vi "Emballage_BDD check code lu.vi"(2 "error in":errorcluster caption="entrée d'erreur", 3 "n° lot à scanner":string="0808", 4 "chaîne lue par le lecteur IN":string="112105740008090004", 5 "tab pcs déjà emballées (histo+actu)":string[](array[string])=["112105740008090009", "112105740008090004", "112105740008090006", "112105740008090007", "112105740008090007R1"], 6 "Quantité du lot de livraison":i32, 16 "n° commande EC":string="R03838/08-01.01.01") -> (9 "error out":errorcluster caption="sortie d'erreur", 13 "offset sur code bar début index":i16=-1, 14 "largeur index":i16=-1, 15 "Date production de la piéce":string, 17 "chaîne lue par le lecteur OUT":string="112105740008090004R1", 18 "Arrêter la série (T)":bool, 19 "Paramètres OK(=> T)":bool)   [LabVIEW 2020]
uses:
  Modules/FS/60_FS_Controles/60_FS_SetGet.ctl
  VG_VerifTests_ModeRetour.vi
  Instance           3 31Saved   Emballage check code lu .vi
panel:
  out "Glissière 2":u8(slide)=100 caption="Identification terminé." scale=0.0..100.0
  out "RETOUR CLIENT":string="1"
  out "tab pcs emballées historique":string[][](array[string])=[["112105740008090004", "01.01.2001 01:01:00", "55", "01234/08-01.01.01", "1", "0"], ["112105740008090006", "01.01.2001 01:01:00", "55", "56789/08-01.01.01", "3", "0"], ["112105740008090007", "01.01.2001 01:01:00", "55", "56789/08-01.01.01", "4", "0"], ["112105740008090007", "01.01.2001 01:01:00", "55", "00123/08-01.01.01", "2", "1"]]
  # "dans historique :\ncolonne 0 = numéro de pièce\ncolonne 1 = date\ncolonne 2 = visa emball\ncolonne 3 = No commande\ncolonne 4 = carton\ncolonne 5 = qtté cmdée ou RC"
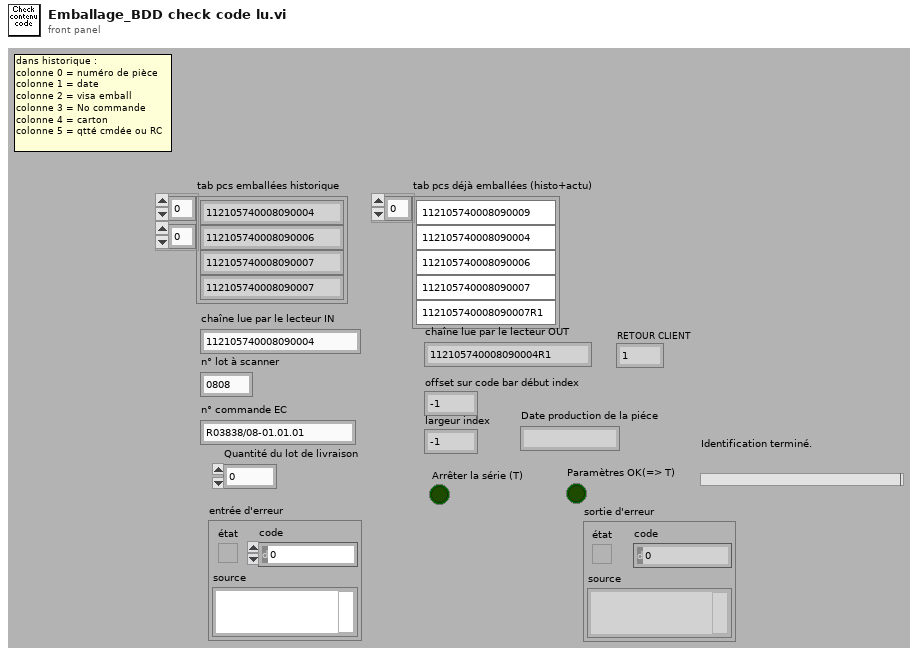
[diagram p1: front panel]
types:
  T1 = typedef "60_FS_SetGet.ctl" = enum16{"set", "get"}
  T2 = typedef "Emballage_BDD_param_Produit.ctl" = cluster{"No_Valve_FAS":string, "suffixe":string, "designation":string, "indice_produit":string, "code_barre_fixe":string, "affiche_code_barre_client":string, "affiche_no_client":string, "Nb_vlve_par_carton":u16, "melange_des_lots_possible":string, "id_article":string, "Indice_Rev":string, "Famille":string, "date":string, "code_barre_fixe_Fin":string, "Longeur_No_Serie":string}
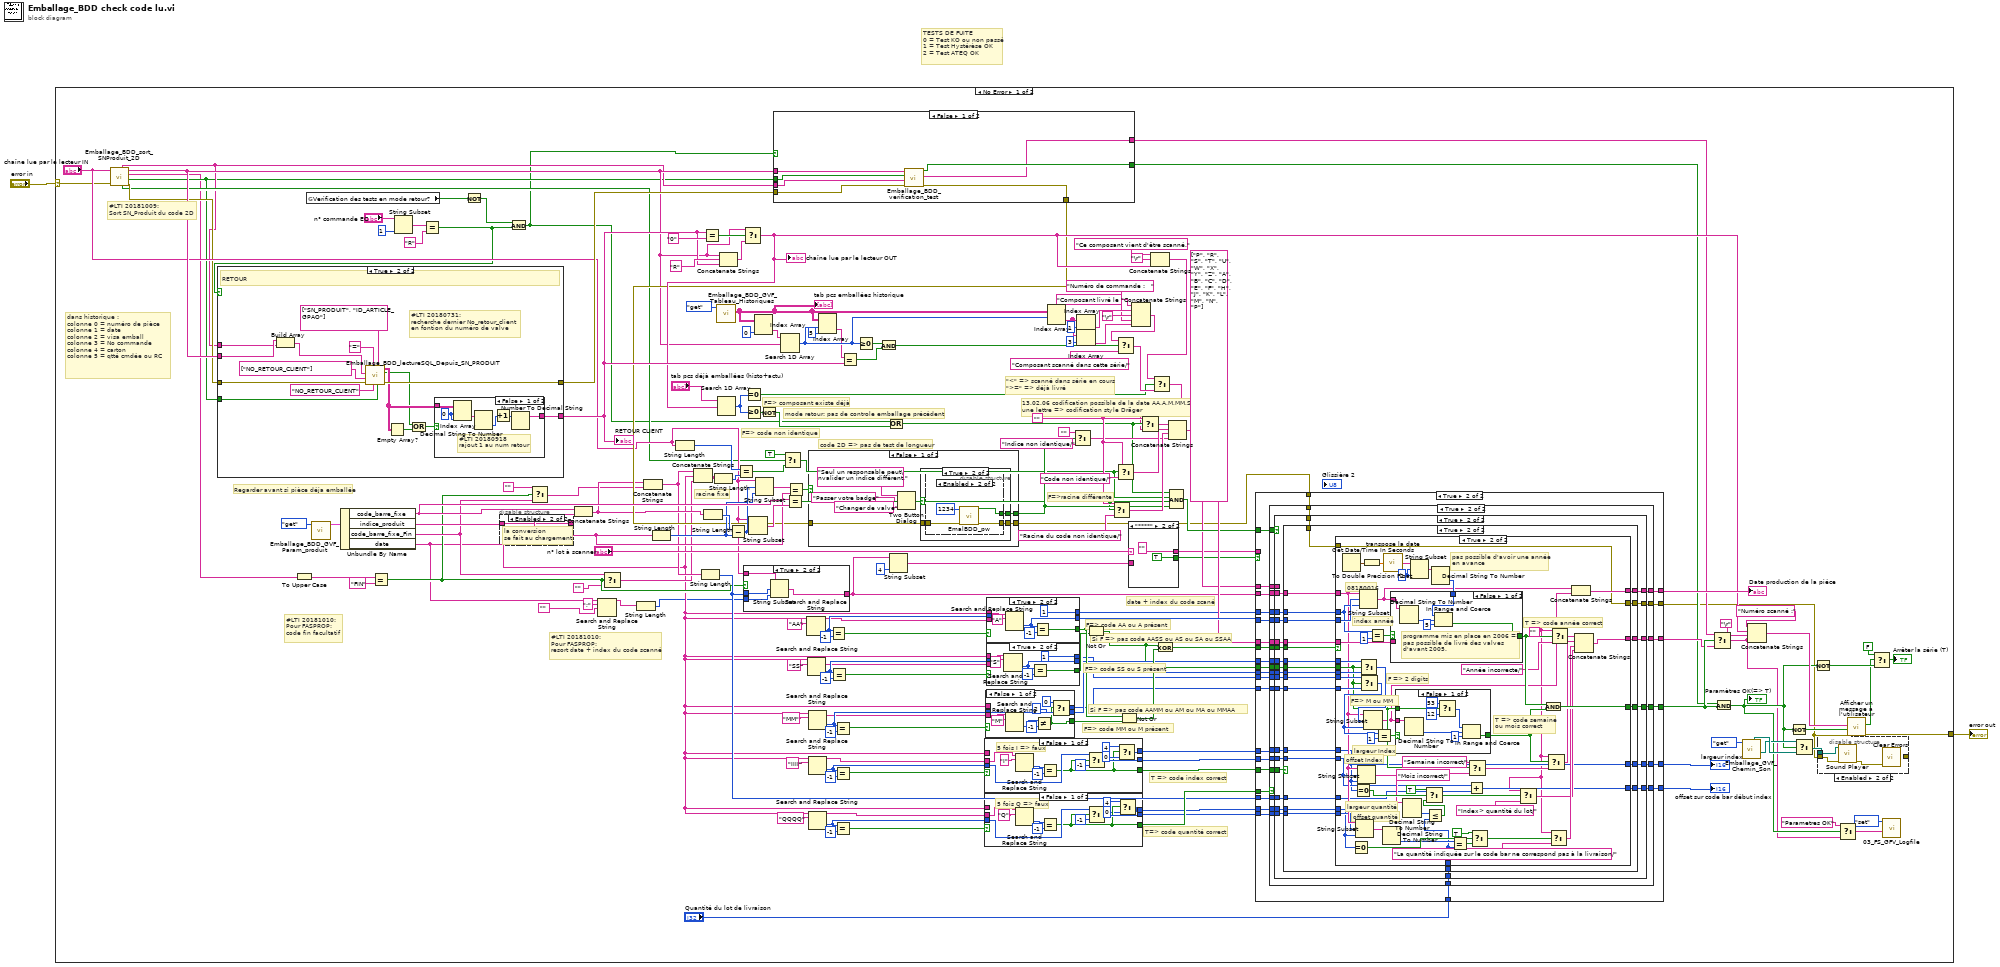
[diagram p0: block diagram]
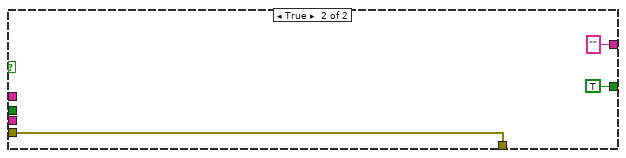
[diagram p2: hidden frame]
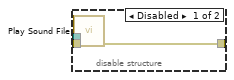
[diagram p3: hidden frame]
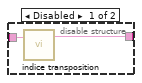
[diagram p4: hidden frame]
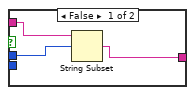
[diagram p5: hidden frame]
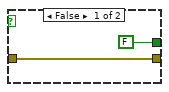
[diagram p6: hidden frame]
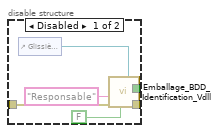
[diagram p7: hidden frame]
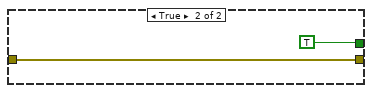
[diagram p8: hidden frame]
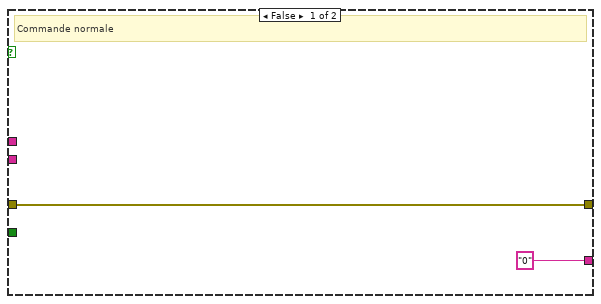
[diagram p9: hidden frame]
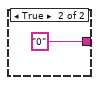
[diagram p10: hidden frame]
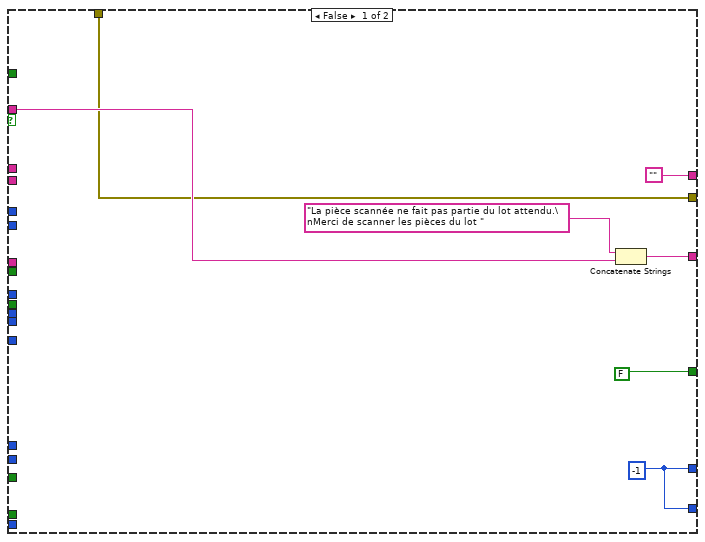
[diagram p11: hidden frame]
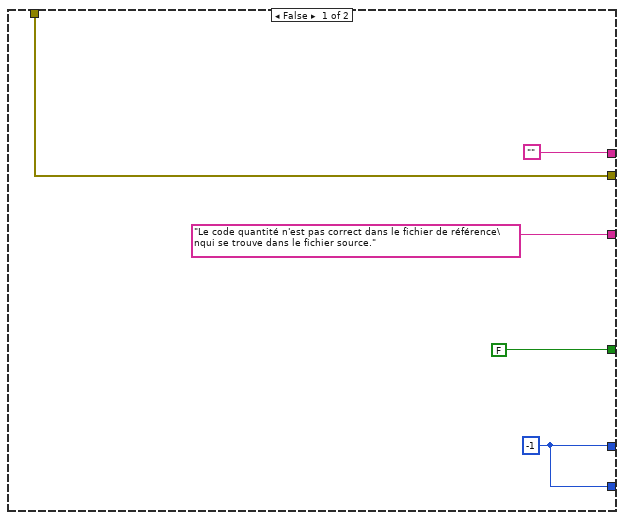
[diagram p12: hidden frame]
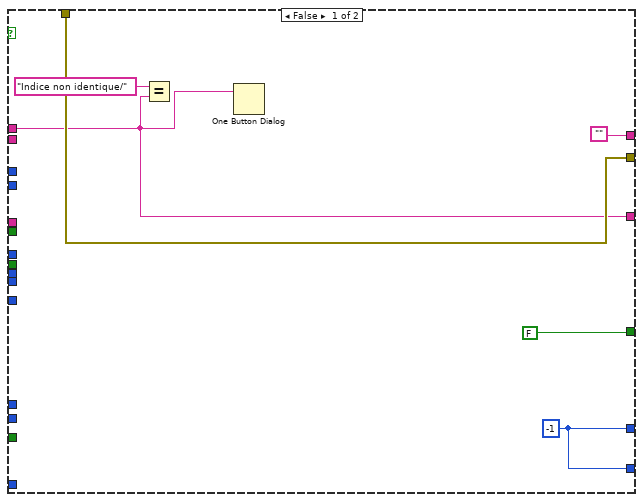
[diagram p13: hidden frame]
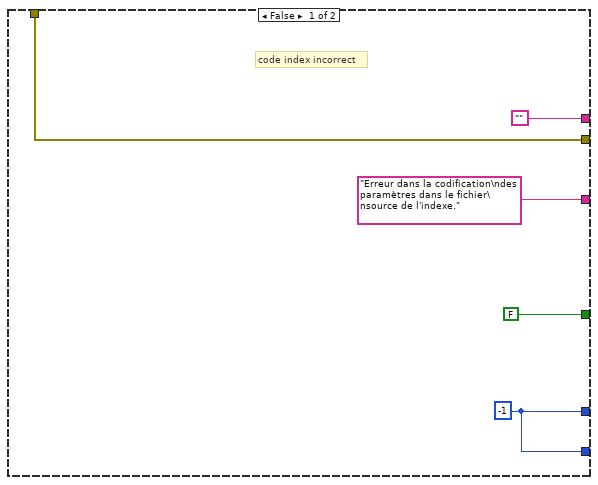
[diagram p14: hidden frame]
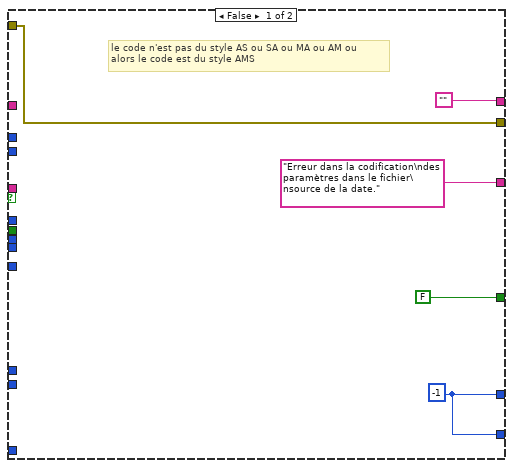
[diagram p15: hidden frame]
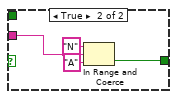
[diagram p16: hidden frame]
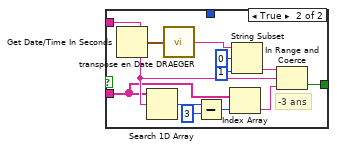
[diagram p17: hidden frame]
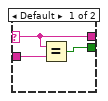
[diagram p18: hidden frame]
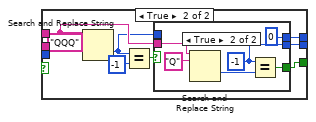
[diagram p19: hidden frame]
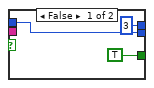
[diagram p20: hidden frame]
diagram:
  # "TESTS DE FUITE\n0 = Test KO ou non passé\n1 = Test Hystérèse OK\n2 = Test ATEQ OK"
  n1 = case shown="No Error" "error in" {
    selector: "error in" -> [w33 w580]
    tunnel: [w70 w580] -> w1
    frame No Error {
      w145 = ""
      # "code 2D => pas de test de longueur"
      # "#LTI 20181010:\nPour FASPROP:\nresort date + index du code scanné"
      # "#LTI 20181010:\nPour FASPROP:\ncode fin facultatif"
      # "#LTI 20181009:\nSort SN_Produit du code 2D"
      # "mode retour: pas de controle emballage précédent"
      # "Regarder avant si pièce déja emballée"
      # "dans historique :\ncolonne 0 = numéro de pièce\ncolonne 1 = date\ncolonne 2 = visa emball\ncolonne 3 = No commande\ncolonne 4 = carton\ncolonne 5 = qtté cmdée ou RC"
      # "\"<\" => scanné dans série en cours\n\">=\" => déjà livré"
      # "T=> code quantité correct"
      # "Si F => pas code AASS ou AS ou SA ou SSAA"
      # "Si F => pas code AAMM ou AM ou MA ou MMAA"
      # "F=> code MM ou M présent"
      # "F=> code SS ou S présent"
      # "F=> code AA ou A présent"
      # "T => code index correct"
      # "13.02.06 codification possible de la date AA,A,M,MM,S,SS\nune lettre => codification style Dräger"
      # "date + index du code scané"
      # "racine fixe"
      # "F=> composant existe déjà"
      # "F=> code non identique"
      # "F=>racine différente"
      n2 = call "Emballage_BDD_sort_SNProduit_2D.vi"("Error in"=w33, "Chaine_Lecteur"="chaîne lue par le lecteur IN") -> ("Error out"=w32:errorcluster, "ID_ARTICLE?"=w12:bool, "emplacement_CodeBarreFinFixe"=w11:string, "SN_PRODUIT"=w36:string, "Code 2D?"=w18:bool, "ID_ARTICLE"=w13:string)  [unwired: 4 in]
      n3 = To Upper Case(1:w11) -> (0:w30:string)
      n4 = global read "VG_VerifTests_ModeRetour.vi" "Verification des tests en mode retour?"() -> (w49:bool)
      n5 = call "Emballage_BDD_GVF_Param_produit.vi"("Énum"=enum16{"set", "get"}."get") -> ("CLS_param_produit"=w43:T2)  [unwired: 7 in, 3 out]
      n6 = Unbundle By Name(w43) -> ("code_barre_fixe"=w64:string, "indice_produit"=w63:string, "code_barre_fixe_Fin"=w26:string, "date"=w23:string)
      n7 = Equal?(x=w30, y="FIN") -> (x = y?=w25:bool)
      n8 = String Subset(string="n° commande EC", length (rest)=1 ("longueur (reste)")) -> (substring=w83:string)  [unwired: 1 in]
      n9 = Equal?(x=w83, y="R" ("expression régulière")) -> (x = y?=w4:bool)
      n10 = case shown="True" w4 {
        tunnel: w36 -> [_ w248]
        tunnel: ["0" ("expression régulière") w247] -> w73
        tunnel: w32 -> [w232 w246]
        tunnel: [w232 w245] -> w69
        tunnel: w13 -> [_ w244]
        tunnel: w12 -> [_ w243]
        frame False {
          # "Commande normale"
        }
        frame True {
          # "#LTI 20180731:\nrecherche dernier No_retour_client\nen fontion du numéro de valve"
          # "RETOUR"
          n11 = Build Array(w248, w244) -> (w235:string[])
          n12 = call "Emballage_BDD_lectureSQL_Depuis_SN_PRODUIT.vi"("ID_ARTICLE?"=w243, "Where (Champs:SN_PRODUIT)"=string[] ["SN_PRODUIT", "ID_ARTICLE_GPAO"], "order by ... DESC"="NO_RETOUR_CLIENT" ("order by"), "Where (Like/=)"="=", "Error in"=w246, "Colonnes"=string[] ["NO_RETOUR_CLIENT"], "Where (Valeur)"=w235) -> ("Error out"=w245:errorcluster, "Erreur de  comunication"=w234:bool, "Donnees"=w239:string[][])  [unwired: 2 in]
          n13 = Empty Array?(array=w239) -> (empty?=w237:bool)
          n14 = Or(x=w234, y=w237) -> (x .or. y?=w238:bool)
          n15 = case shown="False" w238 {
            tunnel: [w249 "0" ("String")] -> w247
            tunnel: w239 -> [w253 _]
            frame False {
              w254 = 0 ("indice (ligne)")
              # "#LTI 20180918\nrajout 1 au num retour"
              n16 = Index Array(array=w253, index (row)=w254, index (col)=w254) -> (element=w252:string)
              n17 = Decimal String To Number(string=w252) -> (number=w251:i32)  [unwired: 2 in, 1 out]
              n18 = Increment(x=w251) -> (x+1=w250:i32)
              n19 = Number To Decimal String(number=w250) -> (decimal integer string=w249:string)  [unwired: 1 in]
            }
            frame True {
            }
          }
        }
      }
      "RETOUR CLIENT" <- w73
      n20 = Not(x=w49) -> (.not. x?=w48:bool)
      n21 = disable-structure shown="Enabled" {
        disable-tunnel: w63 -> [w199 w200]
        disable-tunnel: [w198 w200] -> w59
        frame Disabled {
          n22 = call "indice transposition.vi"("indice entrée"=w199) -> ("indice corrigé"=w198:string)  [unwired: 1 in, 1 out]
        }
        frame Enabled {
          # "la conversion \nse fait au chargement"
        }
      }
      n23 = And(x=w48, y=w4) -> (x .and. y?=w3:bool)
      n24 = Select(t="", s=w25, f=w26) -> (s? t:f=w29:string)
      n25 = Concatenate Strings(w64, w59) -> (w39:string)
      n26 = Search and Replace String(input string=w23, search string=";" ("chaîne recherchée"), replace string="") -> (result string=w20:string)  [unwired: 5 in, 3 out]
      n27 = Select(t=w26, s=w25, f="") -> (s? t:f=w27:string)
      n28 = String Length(string=w20) -> (length=w19:i32)
      n29 = Concatenate Strings(w39, w29) -> (w38:string)
      n30 = String Length(string=w59) -> (length=w61:i32)
      n31 = String Length(string="chaîne lue par le lecteur IN") -> (length=w180:i32)
      n32 = Concatenate Strings(w38, w23, w27) -> (w181:string)
      n33 = String Length(string=w38) -> (length=w37:i32)
      n34 = Equal?(x=w73, y="0" ("chaîne")) -> (x = y?=w74:bool)
      n35 = String Length(string=w39) -> (length=w65:i32)
      n36 = String Length(string=w181) -> (length=w179:i32)
      n37 = call "Emballage_BDD_GVF_Tableau_Historiques.vi"("SetGet"=60_FS_SetGet."get") -> ("Tableau historique OUT"=w42:string[][])  [unwired: 9 in, 1 out]
      "tab pcs emballées historique" <- w42
      n38 = Concatenate Strings(w36, "R" ("chaîne"), w73) -> (w72:string)
      n39 = Subtract(x=w65, y=w61) -> (x-y=w62:i32)
      n40 = Equal?(x=w180, y=w179) -> (x = y?=w17:bool)
      n41 = Select(t=w36, s=w74, f=w72) -> (s? t:f=w71:string)
      "chaîne lue par le lecteur OUT" <- w71
      n42 = Search 1D Array(1D array="tab pcs déjà emballées (histo+actu)", element=w71) -> (index of element=w102:i32)  [unwired: 1 in]
      n43 = case shown="True" w25 {
        tunnel: [w203 w204] -> w95
        tunnel: w37 -> [w202 w206]
        tunnel: "chaîne lue par le lecteur IN" -> [w201 w207]
        tunnel: w19 -> [_ w205]
        frame False {
          n44 = String Subset(string=w201, offset (0)=w202) -> (substring=w203:string)  [unwired: 1 in]
        }
        frame True {
          n45 = String Subset(string=w207, offset (0)=w206, length (rest)=w205) -> (substring=w204:string)
        }
      }
      n46 = Equal To 0?(x=w102) -> (x = 0?=w100:bool)
      n47 = Greater Or Equal To 0?(x=w102) -> (x >= 0?=w149:bool)
      n48 = String Subset(string="chaîne lue par le lecteur IN", length (rest)=w62) -> (substring=w178:string)  [unwired: 1 in]
      n49 = Index Array(array=w42, index (col)=0) -> (element=w103:string[])  [unwired: 1 in]
      n50 = String Subset(string="chaîne lue par le lecteur IN", offset (0)=w62, length (rest)=w61) -> (substring=w60:string)
      n51 = Not(x=w149) -> (.not. x?=w148:bool)
      n52 = case shown="False" w3 {
        tunnel: w36 -> [w188 _]
        tunnel: w69 -> [w187 w189]
        tunnel: [w186 w189] -> w54
        tunnel: [w185 TRUE ("résultat_valve")] -> w50
        tunnel: [w184 "" ("Chaîne explique_probleme")] -> w66
        tunnel: w12 -> [w183 _]
        tunnel: w13 -> [w182 _]
        frame False {
          n53 = call "Emballage_BDD_verification_test.vi"("Error in"=w187, "ID_ARTICLE"=w182, "ID_ARTICLE?"=w183, "Piece_Scanne"=w188) -> ("Error out"=w186:errorcluster, "Chaîne explique_probleme"=w184:string, "résultat_valve"=w185:bool)  [unwired: 5 in]
        }
        frame True {
        }
      }
      n54 = Search 1D Array(1D array=w103, element=w36) -> (index of element=w82:i32)  [unwired: 1 in]
      n55 = Select(t=TRUE ("cas vrai"), s=w18, f=w17) -> (s? t:f=w16:bool)
      n56 = Equal?(x=w64, y=w178) -> (x = y?=w34:bool)
      n57 = Equal?(x=w60, y=w59) -> (x = y?=w55:bool)
      n58 = Search and Replace String(input string=w23, search string="AA") -> (result string=w139:string, offset past replacement=w165:i32)  [unwired: 6 in, 2 out]
      n59 = Search and Replace String(input string=w23, search string="SS") -> (result string=w125:string, offset past replacement=w164:i32)  [unwired: 6 in, 2 out]
      n60 = case shown="False" w55 {
        tunnel: w54 -> [w214 w231]
        tunnel: [w213 w231] -> w53
        tunnel: [w212 TRUE] -> w52
        frame False {
          n61 = Two Button Dialog(message="Seul un responsable peut\nvalider un indice différent.", 1:"Changer de valve" ("Nom du bouton F (\"Annuler\")"), 2:"Passer votre badge" ("Nom du bouton V (\"OK\")")) -> (T button?=w211:bool)
          n62 = case shown="True" w211 {
            tunnel: w214 -> [w216 w219]
            tunnel: [w216 w218] -> w213
            tunnel: [FALSE ("OK") w217] -> w212
            frame False {
            }
            frame True {
              n63 = disable-structure shown="Enabled" {
                disable-tunnel: w219 -> [w222 w228]
                disable-tunnel: [w221 w227] -> w218
                disable-tunnel: [w220 w226] -> w217
                frame Disabled {
                  n64 = control-ref of="Glissière 2"() -> (w225:refnum<vi>)
                  n65 = call "Emballage_BDD_Identification_Vdll.vi"("Glissière"=w225, "lecture seul possible ?"=FALSE, "error in"=w222, "Posage choisi"="Responsable" ("Posage choissi")) -> ("error Out"=w221:errorcluster, "OK"=w220:bool)  [unwired: 3 in, 3 out]
                }
                frame Enabled {
                  n66 = call "EmalBDD_pw.vi"("Error in"=w228, "PWattendu"=u32 1234) -> ("Error Out"=w227:errorcluster, "pwOK?"=w226:bool)  [unwired: 8 in]
                }
              }
            }
          }
        }
        frame True {
        }
      }
      n67 = Search and Replace String(input string=w23, search string="MM") -> (result string=w124:string, offset past replacement=w163:i32)  [unwired: 6 in, 2 out]
      n68 = Search and Replace String(input string=w23, search string="IIII") -> (result string=w140:string, offset past replacement=w134:i32)  [unwired: 6 in, 2 out]
      n69 = Search and Replace String(input string=w23, search string="QQQQ") -> (result string=w132:string, offset past replacement=w131:i32)  [unwired: 6 in, 2 out]
      n70 = Index Array(array=w42, index (row)=w82, index (col)=5) -> (element=w80:string)
      n71 = Equal?(x=w165, y=-1) -> (x = y?=w170:bool)
      n72 = Equal?(x=w164, y=-1) -> (x = y?=w171:bool)
      n73 = Equal?(x=w163, y=-1) -> (x = y?=w169:bool)
      n74 = Equal?(x=w134, y=-1) -> (x = y?=w166:bool)
      n75 = Equal?(x=w131, y=-1) -> (x = y?=w126:bool)
      n76 = Equal?(x=w80, y=w73) -> (x = y?=w79:bool)
      n77 = Greater Or Equal To 0?(x=w82) -> (x >= 0?=w78:bool)
      n78 = And(x=w78, y=w79) -> (x .and. y?=w77:bool)
      n79 = Or(x=w3, y=w148) -> (x .or. y?=w51:bool)
      n80 = String Subset(string=w95, length (rest)=4 ("longueur (reste)")) -> (substring=w90:string)  [unwired: 1 in]
      n81 = case shown="False" w166 {
        tunnel: w23 -> [_ w520]
        tunnel: [w506 w519] -> w135
        tunnel: w140 -> [w512 _]
        tunnel: w134 -> [w511 _]
        tunnel: [w509 w517] -> w133
        tunnel: [w505 w516] -> w128
        frame False {
          # "5 fois I => faux"
          n82 = Search and Replace String(input string=w512, search string="I") -> (offset past replacement=w513:i32)  [unwired: 6 in, 3 out]
          n83 = Equal?(x=w513, y=-1) -> (x = y?=w506:bool)
          n84 = Select(t=w511, s=w506, f=-1) -> (s? t:f=w509:i32)
          n85 = Select(t=4, s=w506, f=0) -> (s? t:f=w505:i32)
        }
        frame True {
          n86 = Search and Replace String(input string=w520, search string="III") -> (offset past replacement=w518:i32)  [unwired: 6 in, 3 out]
          n87 = Equal?(x=w518, y=-1) -> (x = y?=w521:bool)
          n88 = case shown="True" w521 {
            tunnel: w520 -> [_ w531]
            tunnel: [TRUE w529] -> w519
            tunnel: w518 -> [w525 _]
            tunnel: [w525 w528] -> w517
            tunnel: [3 0] -> w516
            frame False {
            }
            frame True {
              w528 = -1
              n89 = Search and Replace String(input string=w531, search string="I") -> (offset past replacement=w530:i32)  [unwired: 6 in, 3 out]
              n90 = Equal?(x=w528, y=w530) -> (x = y?=w529:bool)
            }
          }
        }
      }
      n91 = case shown="False" w126 {
        tunnel: w23 -> [_ w492]
        tunnel: [w480 w491] -> w130
        tunnel: w132 -> [w484 _]
        tunnel: w131 -> [w483 _]
        tunnel: [w481 w489] -> w129
        tunnel: [w477 w488] -> w127
        frame False {
          # "5 fois Q => faux"
          n92 = Search and Replace String(input string=w484, search string="Q") -> (offset past replacement=w485:i32)  [unwired: 6 in, 3 out]
          n93 = Equal?(x=w485, y=-1) -> (x = y?=w480:bool)
          n94 = Select(t=w483, s=w480, f=-1) -> (s? t:f=w481:i32)
          n95 = Select(t=4, s=w480, f=0) -> (s? t:f=w477:i32)
        }
        frame True {
          n96 = Search and Replace String(input string=w492, search string="QQQ") -> (offset past replacement=w490:i32)  [unwired: 6 in, 3 out]
          n97 = Equal?(x=w490, y=-1) -> (x = y?=w493:bool)
          n98 = case shown="True" w493 {
            tunnel: w492 -> [_ w503]
            tunnel: [TRUE w501] -> w491
            tunnel: w490 -> [w497 _]
            tunnel: [w497 w500] -> w489
            tunnel: [3 0] -> w488
            frame False {
            }
            frame True {
              w500 = -1
              n99 = Search and Replace String(input string=w503, search string="Q") -> (offset past replacement=w502:i32)  [unwired: 6 in, 3 out]
              n100 = Equal?(x=w500, y=w502) -> (x = y?=w501:bool)
            }
          }
        }
      }
      n101 = case shown="False" w169 {
        tunnel: w23 -> [_ w547]
        tunnel: [w534 w544] -> w162
        tunnel: [w541 w543] -> w155
        tunnel: w163 -> [w541 _]
        tunnel: [w536 1] -> w152
        tunnel: w124 -> [w537 _]
        frame False {
          n102 = Search and Replace String(input string=w537, search string="M") -> (offset past replacement=w540:i32)  [unwired: 6 in, 3 out]
          n103 = Not Equal?(x=w540, y=-1) -> (x != y?=w534:bool)
          n104 = Select(t=0, s=w534, f=2) -> (s? t:f=w536:i32)
        }
        frame True {
          n105 = Search and Replace String(input string=w547, search string="M") -> (offset past replacement=w543:i32)  [unwired: 6 in, 3 out]
          n106 = Equal?(x=w543, y=-1) -> (x = y?=w544:bool)
        }
      }
      n107 = case shown="True" w171 {
        tunnel: w23 -> [_ w562]
        tunnel: w164 -> [w556 _]
        tunnel: [w556 w559] -> w156
        tunnel: [w548 w558] -> w160
        tunnel: [w551 1] -> w153
        tunnel: w125 -> [w552 _]
        frame False {
          n108 = Search and Replace String(input string=w552, search string="S") -> (offset past replacement=w553:i32)  [unwired: 6 in, 3 out]
          n109 = Not Equal?(x=w553, y=-1) -> (x != y?=w548:bool)
          n110 = Select(t=0, s=w548, f=2) -> (s? t:f=w551:i32)
        }
        frame True {
          n111 = Search and Replace String(input string=w562, search string="S") -> (offset past replacement=w559:i32)  [unwired: 6 in, 3 out]
          n112 = Equal?(x=w559, y=-1) -> (x = y?=w558:bool)
        }
      }
      n113 = case shown="True" w170 {
        tunnel: w23 -> [_ w576]
        tunnel: w165 -> [w571 _]
        tunnel: [w571 w574] -> w157
        tunnel: [w563 w573] -> w161
        tunnel: [w566 1] -> w40
        tunnel: w139 -> [w569 _]
        frame False {
          n114 = Search and Replace String(input string=w569, search string="A") -> (offset past replacement=w567:i32)  [unwired: 6 in, 3 out]
          n115 = Not Equal?(x=w567, y=-1) -> (x != y?=w563:bool)
          n116 = Select(t=0, s=w563, f=2) -> (s? t:f=w566:i32)
        }
        frame True {
          n117 = Search and Replace String(input string=w576, search string="A") -> (offset past replacement=w574:i32)  [unwired: 6 in, 3 out]
          n118 = Equal?(x=w574, y=-1) -> (x = y?=w573:bool)
        }
      }
      n119 = Index Array(array=w42, index (row)=w82) -> (element=w105:string[])  [unwired: 1 in]
      n120 = Select(t="", s=w52, f="Indice non identique/") -> (s? t:f=w56:string)
      n121 = Index Array(array=w105, index=1) -> (element=w108:string)
      n122 = Index Array(array=w105, index=3) -> (element=w89:string)
      n123 = Not Or(1:w160, 2:w161) -> (0:w154:bool)
      n124 = Select(t=w145, s=w34, f="Racine du code non identique/") -> (s? t:f=w142:string)
      n125 = Select(t=w145, s=w16, f="Code non identique/") -> (s? t:f=w143:string)
      n126 = Not Or(1:w162, 2:w161) -> (0:w159:bool)
      n127 = case shown="\"****\"" "n° lot à scanner" {
        selector: "n° lot à scanner" -> [w472 _]
        tunnel: [w474 TRUE] -> w93
        tunnel: [w472 "" ("n° lot à scanner")] -> w92
        tunnel: w90 -> [w473 _]
        frame Default {
          n128 = Equal?(x=w472, y=w473) -> (x = y?=w474:bool)
        }
        frame "****" {
        }
      }
      n129 = Concatenate Strings("Composant livré le ", w108, "\r", "Numéro de commande :   ", w89) -> (w107:string)
      n130 = Select(t=w107, s=w77, f="Composant scanné dans cette série/") -> (s? t:f=w101:string)
      n131 = Concatenate Strings("Ce composant vient d'être scanné.", "\r", w71) -> (w98:string)
      n132 = Select(t=w98, s=w100, f=w101) -> (s? t:f=w14:string)
      n133 = Select(t=w145, s=w51, f=w14) -> (s? t:f=w144:string)
      n134 = Exclusive Or(1:w159, 2:w154) -> (0:w158:bool)
      n135 = Concatenate Strings(w144, w143, w142, w56) -> (w141:string)
      n136 = Compound Arithmetic op=AND(w51, w16, w34, w52) -> (w150:bool)
      n137 = case shown="True" w93 {
        tunnel: w158 -> [_ w289]
        tunnel: w157 -> [_ w288]
        tunnel: w40 -> [_ w287]
        tunnel: w156 -> [_ w286]
        tunnel: w155 -> [_ w285]
        tunnel: w154 -> [_ w284]
        tunnel: w153 -> [_ w283]
        tunnel: w152 -> [_ w282]
        tunnel: string[] ["P", "R", "S", "T", "U", "W", "X", "Y", "Z", "A", "B", "C", "D", "E", "F", "H", "J", "K", "L", "M", "N", "P"] -> [_ w281]
        tunnel: w150 -> [_ w280]
        tunnel: w141 -> [_ w279]
        tunnel: "Quantité du lot de livraison" -> [_ w278]
        tunnel: w135 -> [_ w277]
        tunnel: w133 -> [_ w276]
        tunnel: w130 -> [_ w275]
        tunnel: w129 -> [_ w274]
        tunnel: w128 -> [_ w273]
        tunnel: w127 -> [_ w272]
        tunnel: w37 -> [_ w271]
        tunnel: [w260 w270] -> w123
        tunnel: [w260 w269] -> w122
        tunnel: [w259 w268] -> w67
        tunnel: ["" w267] -> w113
        tunnel: [FALSE w266] -> w68
        tunnel: w95 -> [_ w265]
        tunnel: w92 -> [w257 _]
        tunnel: w53 -> [w256 w264]
        tunnel: [w256 w263] -> w5
        frame False {
          w260 = -1
          n138 = Concatenate Strings("La pièce scannée ne fait pas partie du lot attendu.\nMerci de scanner les pièces du lot ", w257) -> (w259:string)
        }
        frame True {
          n139 = case shown="True" w275 {
            tunnel: w277 -> [_ w320]
            tunnel: w289 -> [_ w319]
            tunnel: w288 -> [_ w318]
            tunnel: w287 -> [_ w317]
            tunnel: w286 -> [_ w316]
            tunnel: w285 -> [_ w315]
            tunnel: w284 -> [_ w314]
            tunnel: w283 -> [_ w313]
            tunnel: w282 -> [_ w312]
            tunnel: w265 -> [_ w311]
            tunnel: w281 -> [_ w310]
            tunnel: w280 -> [_ w309]
            tunnel: w279 -> [_ w308]
            tunnel: ["Le code quantité n'est pas correct dans le fichier de référence\nqui se trouve dans le fichier source." w307] -> w268
            tunnel: [FALSE w306] -> w266
            tunnel: w278 -> [_ w305]
            tunnel: w276 -> [_ w304]
            tunnel: w274 -> [_ w303]
            tunnel: w273 -> [_ w302]
            tunnel: w272 -> [_ w301]
            tunnel: ["" w300] -> w267
            tunnel: w271 -> [_ w299]
            tunnel: [w291 w298] -> w270
            tunnel: [w291 w297] -> w269
            tunnel: w264 -> [w290 w296]
            tunnel: [w290 w295] -> w263
            frame False {
              w291 = -1
            }
            frame True {
              n140 = case shown="True" w309 {
                tunnel: w320 -> [_ w350]
                tunnel: w319 -> [_ w349]
                tunnel: w318 -> [_ w348]
                tunnel: w317 -> [_ w347]
                tunnel: w316 -> [_ w346]
                tunnel: w315 -> [_ w345]
                tunnel: w314 -> [_ w344]
                tunnel: w313 -> [_ w343]
                tunnel: w312 -> [_ w342]
                tunnel: w311 -> [_ w341]
                tunnel: w310 -> [_ w340]
                tunnel: w308 -> [w321 _]
                tunnel: [w321 w338] -> w307
                tunnel: [FALSE w339] -> w306
                tunnel: w305 -> [_ w337]
                tunnel: w304 -> [_ w336]
                tunnel: w303 -> [_ w335]
                tunnel: w302 -> [_ w334]
                tunnel: w301 -> [_ w333]
                tunnel: ["" w332] -> w300
                tunnel: w299 -> [_ w331]
                tunnel: [w325 w330] -> w298
                tunnel: [w325 w329] -> w297
                tunnel: w296 -> [w323 w328]
                tunnel: [w323 w327] -> w295
                frame False {
                  w325 = -1
                  n141 = Equal?(x="Indice non identique/", y=w321) -> ()  [unwired: 1 out]
                  n142 = One Button Dialog(message=w321) -> ()  [unwired: 1 in, 1 out]
                }
                frame True {
                  n143 = case shown="True" w350 {
                    tunnel: w349 -> [_ w378]
                    tunnel: w348 -> [_ w377]
                    tunnel: w347 -> [_ w376]
                    tunnel: w346 -> [_ w375]
                    tunnel: w345 -> [_ w374]
                    tunnel: w344 -> [_ w373]
                    tunnel: w343 -> [_ w372]
                    tunnel: w342 -> [_ w371]
                    tunnel: w341 -> [_ w370]
                    tunnel: w340 -> [_ w369]
                    tunnel: [FALSE w368] -> w339
                    tunnel: ["Erreur dans la codification\ndes paramètres dans le fichier\nsource de l'indexe." w367] -> w338
                    tunnel: w337 -> [_ w366]
                    tunnel: w336 -> [_ w365]
                    tunnel: w335 -> [_ w364]
                    tunnel: w334 -> [_ w363]
                    tunnel: w333 -> [_ w362]
                    tunnel: ["" w361] -> w332
                    tunnel: w331 -> [_ w360]
                    tunnel: [w352 w359] -> w330
                    tunnel: [w352 w358] -> w329
                    tunnel: w328 -> [w351 w357]
                    tunnel: [w351 w356] -> w327
                    frame False {
                      w352 = -1
                      # "code index incorrect"
                    }
                    frame True {
                      n144 = case shown="True" w378 {
                        tunnel: w377 -> [_ w438]
                        tunnel: w376 -> [_ w430]
                        tunnel: w375 -> [_ w442]
                        tunnel: w374 -> [_ w441]
                        tunnel: w373 -> [_ w414]
                        tunnel: w372 -> [_ w440]
                        tunnel: w371 -> [_ w439]
                        tunnel: w370 -> [_ w410]
                        tunnel: w369 -> [_ w428]
                        tunnel: [FALSE w422] -> w368
                        tunnel: ["Erreur dans la codification\ndes paramètres dans le fichier\nsource de la date." w418] -> w367
                        tunnel: w366 -> [_ w397]
                        tunnel: w365 -> [_ w389]
                        tunnel: w364 -> [_ w409]
                        tunnel: w363 -> [_ w386]
                        tunnel: w362 -> [_ w408]
                        tunnel: ["" w390] -> w361
                        tunnel: w360 -> [_ w388]
                        tunnel: [w380 w387] -> w359
                        tunnel: [w380 w386] -> w358
                        tunnel: w357 -> [w379 w385]
                        tunnel: [w379 w385] -> w356
                        frame False {
                          w380 = -1
                          # "le code n'est pas du style AS ou SA ou MA ou AM ou\nalors le code est du style AMS"
                        }
                        frame True {
                          w384 = ""
                          w435 = 2
                          # "08180016"
                          # "largeur quantité"
                          # "largeur Index"
                          # "offset quantité"
                          # "offset Index"
                          # "T => code semaine\nou mois correct"
                          # "pas possible d'avoir une année\nen avance"
                          # "T => code année correct"
                          # "F=> M ou MM"
                          # "F => 2 digits"
                          # "index année"
                          n145 = Get Date/Time In Seconds() -> (seconds since 1Jan1904=w436:timestamp)
                          n146 = Equal To 0?(x=w408) -> (x = 0?=w407:bool)
                          n147 = Equal To 0?(x=w386) -> (x = 0?=w401:bool)
                          n148 = String Subset(string=w410, offset (0)=w409, length (rest)=w408) -> (substring=w403:string)
                          n149 = String Subset(string=w410, offset (0)=w389, length (rest)=w386) -> (substring=w399:string)
                          n150 = String Subset(string=w410, offset (0)=w438, length (rest)=w430) -> (substring=w392:string)
                          n151 = Select(t=w442, s=w414, f=w441) -> (s? t:f=w427:i32)
                          n152 = Select(t=w440, s=w414, f=w439) -> (s? t:f=w425:i32)
                          n153 = To Double Precision Float(number=w436) -> (double precision float=w437:dbl)
                          n154 = String Subset(string=w410, offset (0)=w427, length (rest)=w425) -> (substring=w391:string)
                          n155 = Equal?(x=w430, y=1) -> (x = y?=w429:bool)
                          n156 = Equal?(x=w425, y=1) -> (x = y?=w424:bool)
                          n157 = Decimal String To Number(string=w403) -> (number=w402:i32)  [unwired: 2 in, 1 out]
                          n158 = call "transpose la date.vi"("date a partir du 1 janvier 1904"=w437) -> ("Date:Semaine/année"=w434:string)
                          n159 = case shown="False" w424 {
                            tunnel: w391 -> [w450 w454]
                            tunnel: w414 -> [w446 _]
                            tunnel: [w443 w451] -> w420
                            frame False {
                              n160 = Decimal String To Number(string=w450) -> (number=w449:i32)  [unwired: 2 in, 1 out]
                              n161 = Select(t=53, s=w446, f=12) -> (s? t:f=w447:i32)
                              n162 = In Range and Coerce(upper limit=w447, x=w449, lower limit=1) -> (In Range?=w443:bool)  [unwired: 1 out]
                            }
                            frame True {
                              n163 = In Range and Coerce(upper limit="N", x=w454, lower limit="A") -> (In Range?=w451:bool)  [unwired: 1 out]
                            }
                          }
                          n164 = Decimal String To Number(string=w399) -> (number=w398:i32)  [unwired: 2 in, 1 out]
                          n165 = String Subset(string=w434, offset (0)=w435, length (rest)=w435) -> (substring=w433:string)
                          n166 = Less Or Equal?(x=w398, y=w397) -> (x <= y?=w396:bool)
                          n167 = Select(t=TRUE, s=w401, f=w396) -> (s? t:f=w395:bool)
                          n168 = Decimal String To Number(string=w433) -> (number=w432:i32)  [unwired: 2 in, 1 out]
                          n169 = case shown="False" w429 {
                            tunnel: w392 -> [w459 w466]
                            tunnel: w432 -> [w456 _]
                            tunnel: [w455 w467] -> w423
                            tunnel: w428 -> [_ w462]
                            frame False {
                              # "programme mis en place en 2006 =>\npas possible de livré des valves\nd'avant 2005."
                              n170 = Decimal String To Number(string=w459) -> (number=w458:i32)  [unwired: 2 in, 1 out]
                              n171 = In Range and Coerce(upper limit=w456, x=w458, lower limit=5) -> (In Range?=w455:bool)  [unwired: 1 out]
                            }
                            frame True {
                              # "-3 ans"
                              n172 = Get Date/Time In Seconds() -> (seconds since 1Jan1904=w460:timestamp)
                              n173 = Search 1D Array(1D array=w462, element=w466) -> (index of element=w465:i32)  [unwired: 1 in]
                              n174 = call "transpose en Date DRAEGER.vi"("horodatage"=w460) -> ("Date Dräger"=w469:string)
                              n175 = Subtract(x=w465, y=3) -> (x-y=w463:i32)
                              n176 = Index Array(array=w462, index=w463) -> (element=w461:string)
                              n177 = String Subset(string=w469, offset (0)=0, length (rest)=1) -> (substring=w468:string)
                              n178 = In Range and Coerce(upper limit=w468, x=w466, lower limit=w461) -> (In Range?=w467:bool)  [unwired: 1 out]
                            }
                          }
                          n179 = Equal?(x=w402, y=w397) -> (x = y?=w404:bool)
                          n180 = Add(x=w389, y=w388) -> (x+y=w387:i32)
                          n181 = Select(t="Semaine incorrect/", s=w414, f="Mois incorrect/") -> (s? t:f=w417:string)
                          n182 = Select(t=TRUE, s=w407, f=w404) -> (s? t:f=w406:bool)
                          n183 = Select(t=w384, s=w395, f="Index> quantité du lot/") -> (s? t:f=w393:string)
                          n184 = And(x=w423, y=w420) -> (x .and. y?=w422:bool)
                          n185 = Select(t=w384, s=w420, f=w417) -> (s? t:f=w419:string)
                          n186 = Select(t=w384, s=w406, f="La quantité indiquée sur le code bar ne correspond pas à la livraison/") -> (s? t:f=w411:string)
                          n187 = Select(t=w384, s=w423, f="Année incorrecte/") -> (s? t:f=w421:string)
                          n188 = Concatenate Strings(w392, w391) -> (w390:string)
                          n189 = Concatenate Strings(w421, w419, w411, w393) -> (w418:string)
                        }
                      }
                    }
                  }
                }
              }
            }
          }
        }
      }
      "Date production de la piéce" <- w113
      "offset sur code bar début index" <- w123
      "largeur index" <- w122
      n190 = Select(t=w66, s=w68, f=w67) -> (s? t:f=w6:string)
      n191 = And(x=w50, y=w68) -> (x .and. y?=w7:bool)
      "Paramètres OK(=> T)" <- w7
      n192 = call "Emballage_GVF_Chemin_Son.vi"("Énum"=enum16{"get", "set"}."get") -> ("Chemin lazer.WAV"=w46:path, "Chemin Utopia - Erreur.WAV"=w47:path)  [unwired: 6 in, 3 out]
      n193 = Concatenate Strings("Numéro scanné :", w71, "\r", w6) -> (w116:string)
      n194 = Not(x=w7) -> (.not. x?=w121:bool)
      n195 = Select(t=w46, s=w7, f=w47) -> (s? t:f=w96:path)
      n196 = Not(x=w7) -> (.not. x?=w120:bool)
      n197 = disable-structure shown="Enabled" {
        disable-tunnel: w96 -> [w194 w196]
        disable-tunnel: w5 -> [w193 w197]
        disable-tunnel: [w192 _] -> _
        frame Disabled {
          n198 = call <vilib>:"Play Sound File.vi"("error in (no error)"=w193, "path"=w194) -> ("error out"=w192:errorcluster)  [unwired: 8 in, 1 out]
        }
        frame Enabled {
          n199 = call "Sound Player.vi"("Error in"=w197, "path"=w196) -> ("Error out"=w195:errorcluster)  [unwired: 9 in]
          n200 = call <vilib>:"Clear Errors.vi"("error in (no error)"=w195) -> ()  [unwired: 5 in, 2 out]
        }
      }
      n201 = Select(t="Parametres OK", s=w7, f=w6) -> (s? t:f=w9:string)
      n202 = call "Afficher un message à l'utilisateur"("error in (no error)"=w5, "Enable"=w121, "Message"=w116) -> ("error out"=w70:errorcluster, "Continuer"=w117:bool)  [unwired: 7 in]
      n203 = Select(t=FALSE, s=w117, f=w120) -> (s? t:f=→"Arrêter la série (T)":bool)
      n204 = call "03_FS_GFV_Logfile.vi"("Chaîne"=w9, "States"=60_FS_SetGet."set") -> ()  [unwired: 8 in, 2 out]
    }
    frame Error {
      n205 = call "03_FS_GFV_Logfile.vi"("Chaîne"="erreur avant check_code_lu", "States"=60_FS_SetGet."set") -> ()  [unwired: 8 in, 2 out]
    }
  }
  "error out" <- w1
